vi "Retrieve L (FPGA).vi"(10 "Matrix In":fxp<+/-,48,48>[](array[numeric])=[0.0, 0.0, 0.0, 0.0, 0.0, 0.0, 0.0, 0.0, 0.0]) -> (3 "L":fxp<+,64,57>[](array[numeric]) format="%.25g")   [LabVIEW 2014]
uses:
  <vilib>/rvi/FXPMathLib/FxpDiv/subVIs/nifxpmath_Div_SimConfig.ctl
  <vilib>/rvi/FXPMathLib/FxpSqrt/subVIs/nifxpmath_Sqrt_SimConfig.ctl
  <vilib>/fxp/LVFixedPointOverflowPolicyTypeDef.ctl
  <vilib>/rvi/Emulation/niFpgaGetClockAttributes.vi
  <vilib>/rvi/Emulation/niFpgaSctlEmulationGetInTimedLoop.vi
  <vilib>/rvi/Emulation/niFpgaEmulationReportErrorSimple.vi
  <vilib>/rvi/Emulation/niFpgaCriticalErrorInLSC.vi
  <vilib>/rvi/FXPMathLib/FxpDiv/simVIs/DllFxpDivTemp_sub.vi
  <vilib>/rvi/FXPMathLib/FxpSqrt/simVIs/DllSqrtTemp_sub.vi
  <vilib>/rvi/FXPMathLib/FxpMul/XNode/nifxpmath_Multiplier.xnode
  <vilib>/rvi/FXPMathLib/FxpSub/XNode/nifxpmath_Sub.xnode
  <vilib>/rvi/FXPMathLib/FxpDiv/XNode/nifxpmath_Div.xnode
  <vilib>/rvi/FXPMathLib/FxpSqrt/XNode/nifxpmath_Sqrt.xnode
  <vilib>/rvi/FXPMathLib/sim/FxpSim.dll
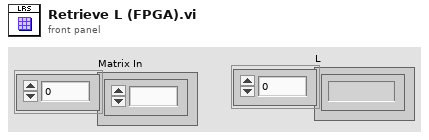
[diagram p1: front panel]
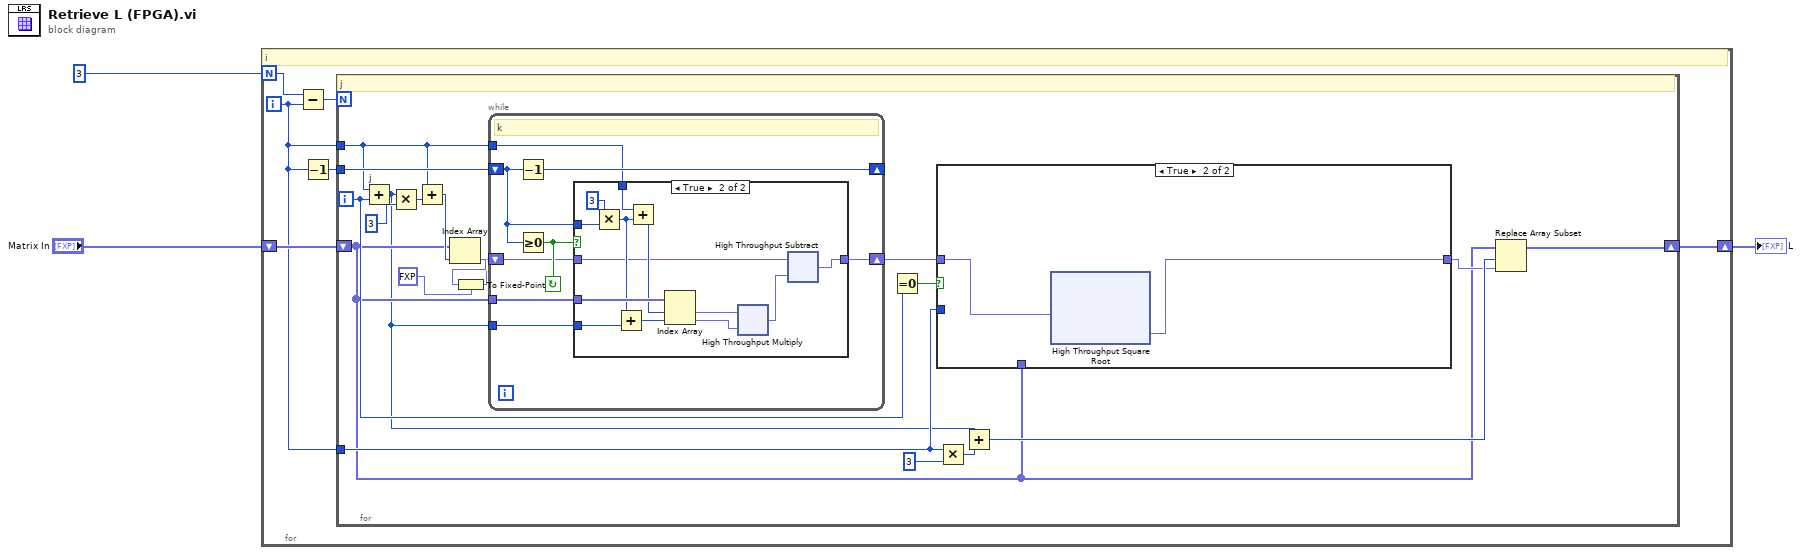
[diagram p0: block diagram]
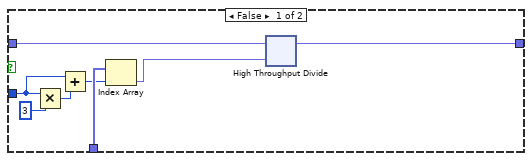
[diagram p2: hidden frame]
diagram:
  n1 = for {
    N: 3 -> [w9]
    shift-right: [w4] -> w1
    shift-left: "Matrix In" -> [w6]
    i -> [w5]
    # "i"
    n2 = Subtract(x=w9, y=w5) -> (x-y=w8:i32)
    n3 = Decrement(x=w5) -> (x-1=w7:i32)
    n4 = for {
      N: w8 -> [_]
      tunnel: w7 -> [w28]
      tunnel: w5 -> [w25]
      tunnel: w5 -> [w15]
      shift-right: [w18] -> w4
      shift-left: w6 -> [w14]
      i -> [w21]
      # "j"
      n5 = Add "j"(x=w25, y=w21) -> (x+y=w13:i32)
      n6 = Multiply(x=w13, y=3) -> (x*y=w24:i32)
      n7 = Add(x=w25, y=w24) -> (x+y=w26:i32)
      n8 = Index Array(array=w14, index=w26) -> (element=w12:fxp<+/-,48,48>)
      n9 = To Fixed-Point(fixed-point type=fxp<+,64,57> 0.0 ("x-y"), number=w12) -> (fixed-point=w11:fxp<+,64,57>)
      n10 = while {
        shift-right: [w94] -> _
        shift-left: w28 -> [w90]
        shift-right: [w89] -> w22
        shift-left: w11 -> [w93]
        tunnel: w14 -> [w92]
        tunnel: w25 -> [w91]
        tunnel: w13 -> [w88]
        stop <- w95 continue-if-true
        # "k"
        n11 = Decrement(x=w90) -> (x-1=w94:i32)
        n12 = Greater Or Equal To 0?(x=w90) -> (x >= 0?=w95:bool)
        n13 = case shown="True" w95 {
          tunnel: w93 -> [w96 w100]
          tunnel: w92 -> [_ w109]
          tunnel: w91 -> [_ w97]
          tunnel: w90 -> [_ w108]
          tunnel: [w96 w98] -> w89
          tunnel: w88 -> [_ w105]
          frame False {
          }
          frame True {
            n14 = Multiply(x=3 ("y"), y=w108) -> (x*y=w104:i32)
            n15 = Add(x=w104, y=w105) -> (x+y=w103:i32)
            n16 = Add(x=w97, y=w104) -> (x+y=w106:i32)
            n17 = Index Array(array=w109, index #1=w106, index #2=w103) -> (element #1=w102:fxp<+/-,48,48>, element #2=w101:fxp<+/-,48,48>)
            n18 = xnode ("High Throughput Multiply")("x"=w102, "y"=w101) -> ("x*y"=w99:fxp<+,64,57>)
            n19 = xnode "High Throughput Subtract"("x"=w100, "y"=w99) -> ("x-y"=w98:fxp<+,64,57>)
          }
        }
      }
      n20 = Equal To 0?(x=w21) -> (x = 0?=w23:bool)
      n21 = case shown="True" w23 {
        tunnel: w22 -> [w31 w65]
        tunnel: [w29 w64] -> w16
        tunnel: w15 -> [w34 _]
        tunnel: w14 -> [w33 _]
        frame False {
          n22 = Multiply(x=w34, y=3 ("x")) -> (x*y=w35:i32)
          n23 = Add(x=w34, y=w35) -> (x+y=w32:i32)
          n24 = Index Array(array=w33, index=w32) -> (element=w30:fxp<+/-,48,48>)
          n25 = xnode "High Throughput Divide"("x"=w31, "y"=w30) -> ("x/y"=w29:fxp<+/-,64,57>)
        }
        frame True {
          n26 = xnode "High Throughput Square Root"("x"=w65) -> ("sqrt(x)"=w64:fxp<+,33,29>)
        }
      }
      n27 = Multiply(x=w15, y=3 ("x")) -> (x*y=w19:i32)
      n28 = Add(x=w13, y=w19) -> (x+y=w17:i32)
      n29 = Replace Array Subset(array=w14, new element=w16, index=w17) -> (w18:fxp<+/-,48,48>[])
    }
  }
  "L" <- w1
